vi "XL320_Ping.vi"(8 "error in (no error)":errorcluster, 10 "Motor ID":u8, 11 "VISA Refnum in":refnum<visa-resource-name>) -> (0 "error out":errorcluster, 2 "Motor ID out":u8, 3 "VISA Refnum out":refnum<visa-resource-name>)   [LabVIEW 2017, in "Dynamixel XL320.lvlib"]
uses:
  <instrlib>/Dynamixel XL320 (Drivers instrument)/Dynamixel XL320.lvlib
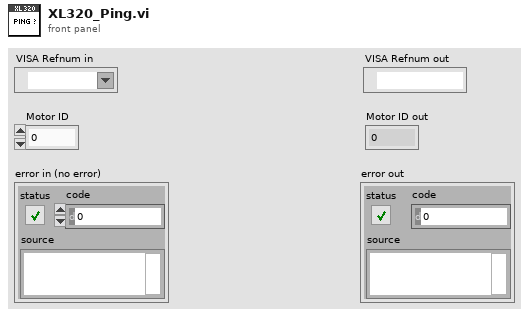
[diagram p1: front panel]
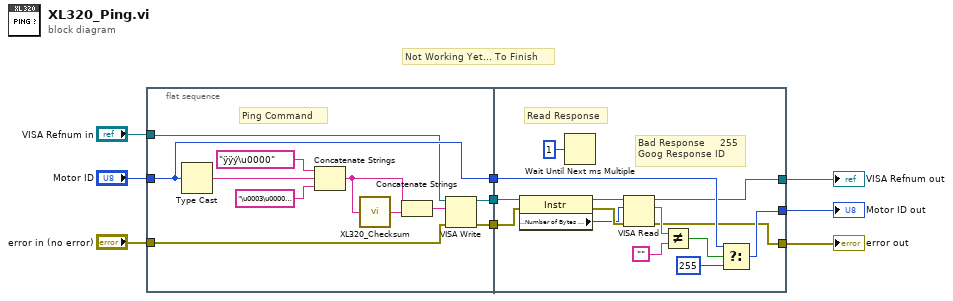
[diagram p0: block diagram]
diagram:
  # "Not Working Yet... To Finish"
  n1 = flat-sequence {
    tunnel: "VISA Refnum in" -> [w13]
    tunnel: [w11] -> w5
    tunnel: "error in (no error)" -> [w12]
    tunnel: "Motor ID" -> [w14]
    tunnel: [w14] -> w4
    tunnel: [w10] -> w3
    tunnel: w5 -> [w28]
    tunnel: w4 -> [w26]
    tunnel: [w25] -> w9
    tunnel: w3 -> [w27]
    tunnel: [w23] -> w2
    tunnel: [w22] -> w1
    frame #0 {
      # "Ping Command"
      n2 = Type Cast(x=w14) -> (*(type *) &x=w17:string)  [unwired: 1 in]
      n3 = Concatenate Strings("ÿÿý\u0000", w17, "\u0003\u0000\u0001") -> (w19:string)
      n4 = call <instrlib>:"XL320_Checksum.vi"("Input String"=w19) -> ("Checksum String"=w18:string)
      n5 = Concatenate Strings(w19, w18) -> (w20:string)
      n6 = VISA Write(VISA resource name=w13, write buffer=w20, error in (no error)=w12) -> (VISA resource name out=w11:refnum<visa-resource-name>, error out=w10:errorcluster)  [unwired: 1 out]
    }
    frame #1 {
      # "Bad Response     255\nGoog Response ID"
      # "Read Response"
      n7 = property class="Instr"(reference=w28, error in=w27) -> (reference out=w32:refnum<visa-resource-name>, error out=w34:errorcluster, "Serial Settings:Number of Bytes at Serial Port"=w33:u32)
      n8 = Wait Until Next ms Multiple(millisecond multiple=u32 1 ("milliseconds to wait")) -> ()  [unwired: 1 out]
      n9 = VISA Read(VISA resource name=w32, byte count=w33, error in (no error)=w34) -> (VISA resource name out=w23:refnum<visa-resource-name>, read buffer=w30:string, error out=w22:errorcluster)  [unwired: 1 out]
      n10 = Not Equal?(x=w30, y="") -> (x != y?=w29:bool)
      n11 = Select(t=w26, s=w29, f=u8 255) -> (s? t:f=w25:u8)
    }
  }
  "error out" <- w1
  "VISA Refnum out" <- w2
  "Motor ID out" <- w9
